vi "Execute.vi"(8 "error in (no error)":errorcluster, 10 "Abstract Producer in":refnum<class "Abstract Producer.lvclass">, 11 "Manage File Response in":refnum<class "Manage File Response.lvclass">) -> (0 "error out":errorcluster, 2 "Abstract Producer out":refnum<class "Abstract Producer.lvclass">, 3 "Manage File Response out":refnum<class "Manage File Response.lvclass">)   [LabVIEW 2020, in "AIM ARINC 664 Engine.lvlib" / "Implementation.lvlib" / "Frame Logging.lvlib" / "Manage File Response.lvclass"]
uses:
  <vilib>/NI/VeriStand Custom Device Messaging/Producer/Abstract Producer/Abstract Producer.lvclass
  Manage File Response.lvclass
  Manage File Response.lvclass/Manage File Response.ctl
  <vilib>/NI/VeriStand Custom Device Messaging/Message/Abstract Response Message/Abstract Response Message.lvclass
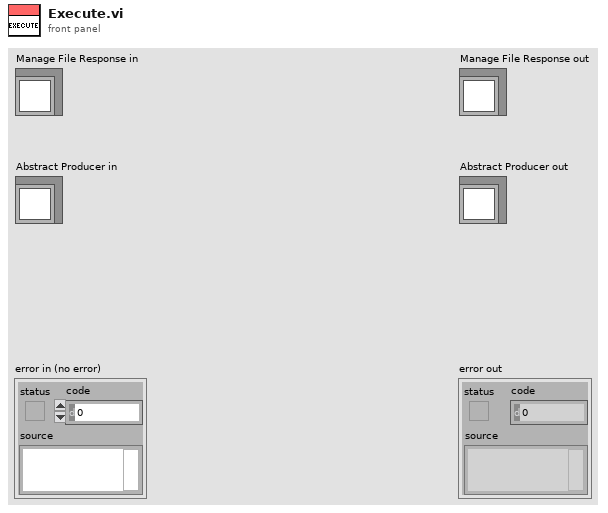
[diagram p1: front panel]
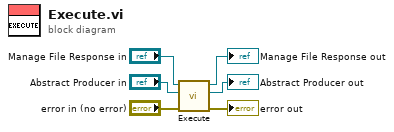
[diagram p0: block diagram]
diagram:
  n1 = call-parent "Execute.vi"("error in (no error)"="error in (no error)", "Abstract Producer in"="Abstract Producer in", "Abstract Response Message in"="Manage File Response in") -> ("error out"=→"error out":errorcluster, "Abstract Producer out"=→"Abstract Producer out":refnum<class "Abstract Producer.lvclass">, "Abstract Response Message out"=→"Manage File Response out":refnum<class "Manage File Response.lvclass">)  [unwired: 6 in]
